vi "pDataBufferToRGBimage.vi"(7 "Draw spots":bool, 8 "error in (no error)":errorcluster, 9 "Spot Radius":dbl=3.0 format="%#_13g", 10 "Img Dst":refnum<image>=refnum, 11 "pDataBuffer":u16[](array[numeric])=array[8192 elements]) -> (0 "error out":errorcluster, 3 "Img Out":refnum<image>)   [LabVIEW 2020]
uses:
  _Globals/Global Controls.vi
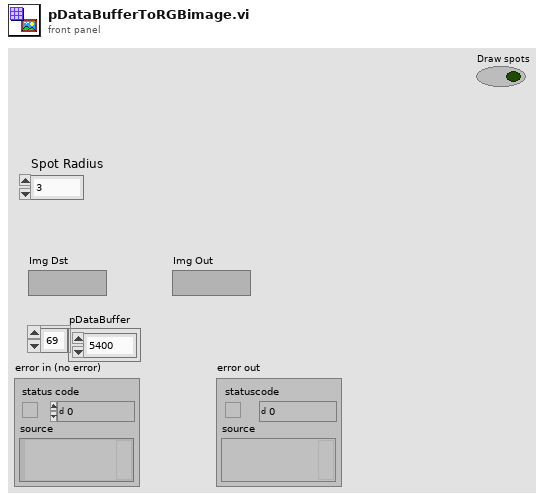
[diagram p1: front panel]
types:
  T1 = typedef "Tweezertron Ctrl Refs.ctl" = cluster{"LSM Settings":refnum<vi>, "iFlex Control":refnum<vi>, "PIFOC Settings":refnum<vi>, "PinSelector":refnum<vi>, "Manlight Controls":refnum<vi>, "Exp Params":refnum<vi>, "Image Thresholds":refnum<vi>, "RevFrame":refnum<vi>, "Spots":refnum<vi>}
  T2 = typedef "Image Thresholds.ctl" = cluster{"Channel A":cluster{u16, u16}, "Channel B":cluster{u16, u16}}
  T3 = typedef "Confocal Controls.ctl" = cluster{"Channel Selection":enum32{"A", "B", "AB"}, "Pixel Count":cluster{"Pixels in X":u32, "Pixels in Y":u32}, "Field Size":dbl, "Frames":u8, "Averaging":bool, "Alignment":cluster{"Course":dbl, "Fine":dbl}, "Scan Mode":bool, "Gain":cluster{"Gain A":u8, "Gain B":u8}, "Enable PMTs":cluster{"A":bool, "B":bool}, "Voltage Range":cluster{"Range A":u16, "Range B":u16}, "Field Size in um":dbl, "MicronsPerPx":dbl, "Multi Frame Count":dbl, "Trigger Mode":dbl, "Real Time Averaging":bool}
  T4 = cluster{"element":u16, "element":u16, "element":u16, "element":u16}[]
  T5 = cluster{"element":u16, "element":u16, "element":u16, "element":u16}[][]
  T6 = typedef "IMAQ Image.ctl" = refnum<image>
  T7 = typedef "SLM Real World to IMAQ Display Transform.ctl" = cluster{"Translation":cluster{"X":dbl, "Y":dbl}, "Scalling":cluster{"xScale":dbl, "yScale":dbl}}
  T8 = typedef "Spots.ctl" = cluster{"Spot Params":T9, "Add Spot":bool, "Remove Spot":bool, "Clear All Spots":bool, "Save Spots":bool, "Generate Spots":bool, "Generate Pattern":string, "load spots":bool}
  T9 = typedef "Spot Params.ctl" = cluster{"Intensity":dbl, "Vortex":dbl, "Phase":dbl, "X":dbl, "Y":dbl, "Z":dbl}[]
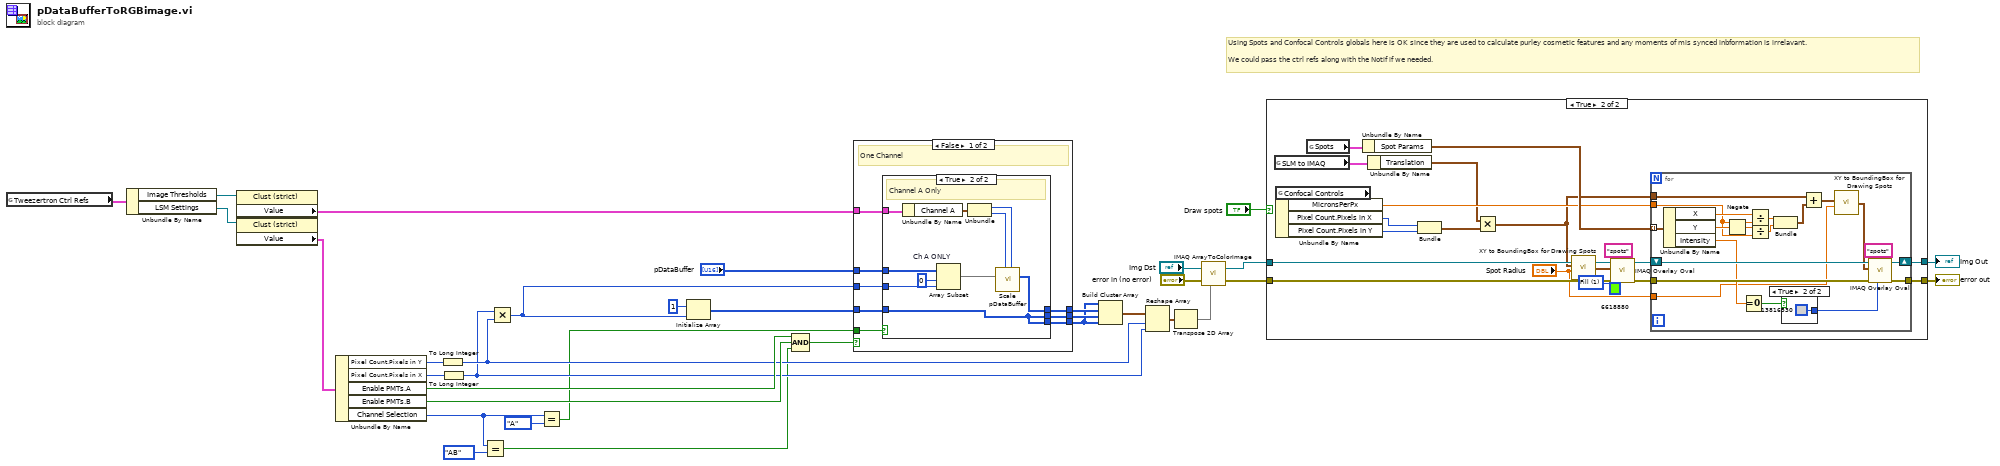
[diagram p0: block diagram]
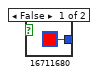
[diagram p3: hidden frame]
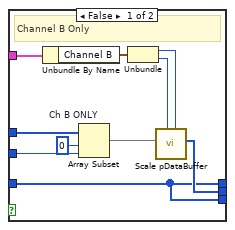
[diagram p4: hidden frame]
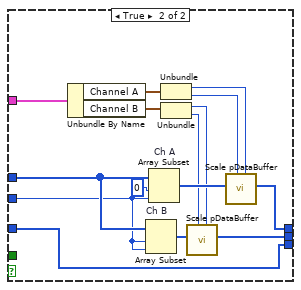
[diagram p5: hidden frame]
diagram:
  # "Using Spots and Confocal Controls globals here is OK since they are used to calculate purley cosmetic features and any moments of mis synced inbformation is irrelavant.\n\nWe could pass the ctrl refs along with the Notif if we needed."
  n1 = global read "Global Controls.vi" "Tweezertron Ctrl Refs"() -> (w9:T1)
  n2 = Unbundle By Name(w9) -> ("Image Thresholds"=w8:refnum<vi>, "LSM Settings"=w6:refnum<vi>)
  n3 = property class="Clust (strict)"(reference=w8) -> ("Value"=w7:T2)  [unwired: 1 in, 2 out]
  n4 = property class="Clust (strict)"(reference=w6) -> ("Value"=w5:T3)  [unwired: 1 in, 2 out]
  n5 = Unbundle By Name(w5) -> ("Pixel Count.Pixels in Y"=w20:u32, "Pixel Count.Pixels in X"=w19:u32, "Enable PMTs.A"=w33:bool, "Enable PMTs.B"=w31:bool, "Channel Selection"=w13:enum32{"A", "B", "AB"})
  n6 = To Long Integer(number=w20) -> (32bit integer=w18:i32)
  n7 = To Long Integer(number=w19) -> (32bit integer=w17:i32)
  n8 = Equal?(x=w13, y=enum32{"A", "B", "AB"}."AB") -> (x = y?=w14:bool)
  n9 = Multiply(x=w17, y=w18) -> (x*y=w10:i32)
  n10 = Equal?(x=w13, y=enum32{"A", "B", "AB"}."A") -> (x = y?=w11:bool)
  n11 = Initialize Array(u16 1 ("element"), w10) -> (w4:u16[])
  n12 = Compound Arithmetic op=AND(w33, w31, w14) -> (w32:bool)
  n13 = case shown="False" w32 {
    tunnel: w4 -> [w42 w63]
    tunnel: [w40 w69] -> w21
    tunnel: [w41 w70] -> w22
    tunnel: "pDataBuffer" -> [w39 w71]
    tunnel: w10 -> [w38 w68]
    tunnel: w7 -> [w37 w67]
    tunnel: w11 -> [w36 _]
    tunnel: [w35 w63] -> w3
    frame False {
      # "One Channel"
      n14 = case shown="True" w36 {
        tunnel: [w43 w55] -> w40
        tunnel: w42 -> [w43 w53]
        tunnel: [w44 w53] -> w41
        tunnel: w39 -> [w50 w60]
        tunnel: w38 -> [w49 w59]
        tunnel: w37 -> [w47 w54]
        tunnel: [w43 w53] -> w35
        frame False {
          # "Channel B Only"
          n15 = Unbundle By Name(w47) -> ("Channel B"=w48:cluster{u16, u16})
          n16 = Array Subset "Ch B ONLY"(array=w50, index=0, length=w49) -> (w51:u16[])
          n17 = Unbundle(w48) -> (w46:u16, w45:u16)
          n18 = call "Scale pDataBuffer.vi"("Min"=w46, "Max"=w45, "pDataBuffer"=w51) -> ("Scaled pDataBuffer"=w44:u16[])  [unwired: 8 in]
        }
        frame True {
          # "Channel A Only"
          n19 = Unbundle By Name(w54) -> ("Channel A"=w58:cluster{u16, u16})
          n20 = Array Subset "Ch A ONLY"(array=w60, index=0, length=w59) -> (w61:u16[])
          n21 = Unbundle(w58) -> (w57:u16, w56:u16)
          n22 = call "Scale pDataBuffer.vi"("Min"=w57, "Max"=w56, "pDataBuffer"=w61) -> ("Scaled pDataBuffer"=w55:u16[])  [unwired: 8 in]
        }
      }
    }
    frame True {
      n23 = Unbundle By Name(w67) -> ("Channel A"=w75:cluster{u16, u16}, "Channel B"=w66:cluster{u16, u16})
      n24 = Array Subset "Ch B"(array=w71, index=w68, length=w68) -> (w72:u16[])
      n25 = Array Subset "Ch A"(array=w71, index=0, length=w68) -> (w76:u16[])
      n26 = Unbundle(w75) -> (w74:u16, w73:u16)
      n27 = Unbundle(w66) -> (w65:u16, w64:u16)
      n28 = call "Scale pDataBuffer.vi"("Min"=w65, "Max"=w64, "pDataBuffer"=w72) -> ("Scaled pDataBuffer"=w70:u16[])  [unwired: 8 in]
      n29 = call "Scale pDataBuffer.vi"("Min"=w74, "Max"=w73, "pDataBuffer"=w76) -> ("Scaled pDataBuffer"=w69:u16[])  [unwired: 8 in]
    }
  }
  n30 = Build Cluster Array(w3, w21, w22, w3) -> (w30:T4)
  n31 = Reshape Array(w30, w18, w17) -> (w2:T5)
  n32 = Transpose 2D Array(2D array=w2) -> (transposed array=w1:T5)
  n33 = call "IMAQ ArrayToColorImage"("Image"="Img Dst", "Image Pixels (U64)"=w1, "error in (no error)"="error in (no error)") -> ("Image Out"=w26:T6, "error out"=w25:errorcluster)  [unwired: 2 in]
  n34 = case shown="True" "Draw spots" {
    tunnel: w26 -> [w79 w100]
    tunnel: w25 -> [w78 w99]
    tunnel: [w78 w93] -> w23
    tunnel: [w79 w96] -> w24
    frame False {
    }
    frame True {
      w85 = u32 1 items=["Frame", "Fill"] ("Drawing Mode (Frame)")
      n35 = global read "Global Controls.vi" "SLM to IMAQ"() -> (w86:T7)
      n36 = global read "Global Controls.vi" "Confocal Controls"() -> (w92:T3)
      n37 = Unbundle By Name(w92) -> ("MicronsPerPx"=w88:dbl, "Pixel Count.Pixels in X"=w84:u32, "Pixel Count.Pixels in Y"=w83:u32)
      n38 = global read "Global Controls.vi" "Spots"() -> (w90:T8)
      n39 = Unbundle By Name(w90) -> ("Spot Params"=w89:T9)
      n40 = Unbundle By Name(w86) -> ("Translation"=w81:cluster{"X":dbl, "Y":dbl})
      n41 = Bundle("Pixels in X"=w84, "Pixels in Y"=w83) -> (w82:cluster{"Pixels in X":u32, "Pixels in Y":u32})  [unwired: 1 in]
      n42 = Multiply(x=w81, y=w82) -> (x*y=w80:cluster{dbl, dbl})
      n43 = call "XY to BoundingBox for Drawing Spots.vi"("Radius"="Spot Radius", "Central Coords"=w80) -> ("Bounding Box"=w91:cluster{dbl, dbl, dbl, dbl})  [unwired: 2 in]
      n44 = call "IMAQ Overlay Oval"("Color"=u32 6618880, "Group"="spots", "error in (no error)"=w99, "Drawing Mode (Frame)"=w85, "Bounding Rectangle"=w91, "Image"=w100) -> ("error out"=w94:errorcluster, "Image Out"=w95:T6)  [unwired: 4 in]
      n45 = for {
        tunnel: w89 -> [w118] mode=indexing
        shift-right: [w117] -> w96
        shift-left: w95 -> [w116]
        tunnel: w94 -> [w115]
        tunnel: [w114] -> w93
        tunnel: w88 -> [w111]
        tunnel: w80 -> [w107]
        tunnel: "Spot Radius" -> [w101]
        n46 = Unbundle By Name(w118) -> ("X"=w113:dbl, "Y"=w112:dbl, "Intensity"=w105:dbl)
        n47 = Negate(x=w112) -> (-x=w102:dbl)
        n48 = Equal To 0?(x=w105) -> (x = 0?=w106:bool)
        n49 = Divide(x=w113, y=w111) -> (x/y=w110:dbl)
        n50 = Divide(x=w102, y=w111) -> (x/y=w109:dbl)
        n51 = Bundle(w110, w109) -> (w108:cluster{dbl, dbl})  [unwired: 1 in]
        n52 = case shown="True" w106 {
          tunnel: [u32 16711680 ("Color") u32 13816530 ("Color")] -> w120
          frame False {
          }
          frame True {
          }
        }
        n53 = Add(x=w107, y=w108) -> (x+y=w104:cluster{dbl, dbl})
        n54 = call "XY to BoundingBox for Drawing Spots.vi"("Radius"=w101, "Central Coords"=w104) -> ("Bounding Box"=w103:cluster{dbl, dbl, dbl, dbl})  [unwired: 2 in]
        n55 = call "IMAQ Overlay Oval"("Color"=w120, "Group"="spots", "error in (no error)"=w115, "Bounding Rectangle"=w103, "Image"=w116) -> ("error out"=w114:errorcluster, "Image Out"=w117:T6)  [unwired: 5 in]
      }
    }
  }
  "Img Out" <- w24
  "error out" <- w23
